vi "Merge Call Library Errors.vi"(4 "Library Call Returned Error":errorcluster, 6 "Error Code":i32(ring) items=["No Error", "mArgsErr", "mZoneErr", "mFullErr"], 8 "error in":errorcluster) -> (0 "error out":errorcluster)   [LabVIEW 2020, in "ase.lvlib" / "ase.lvclass"]
doc: "Combine Call Library Function Node Errors and Error Codes."
uses:
  ase.lvclass
  ase.lvclass/ase.ctl
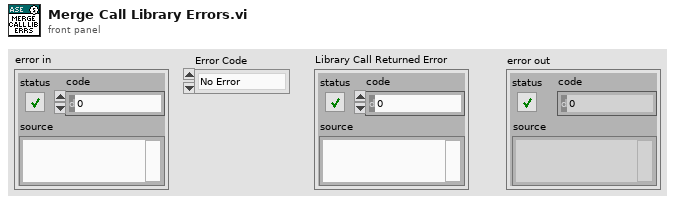
[diagram p1: front panel]
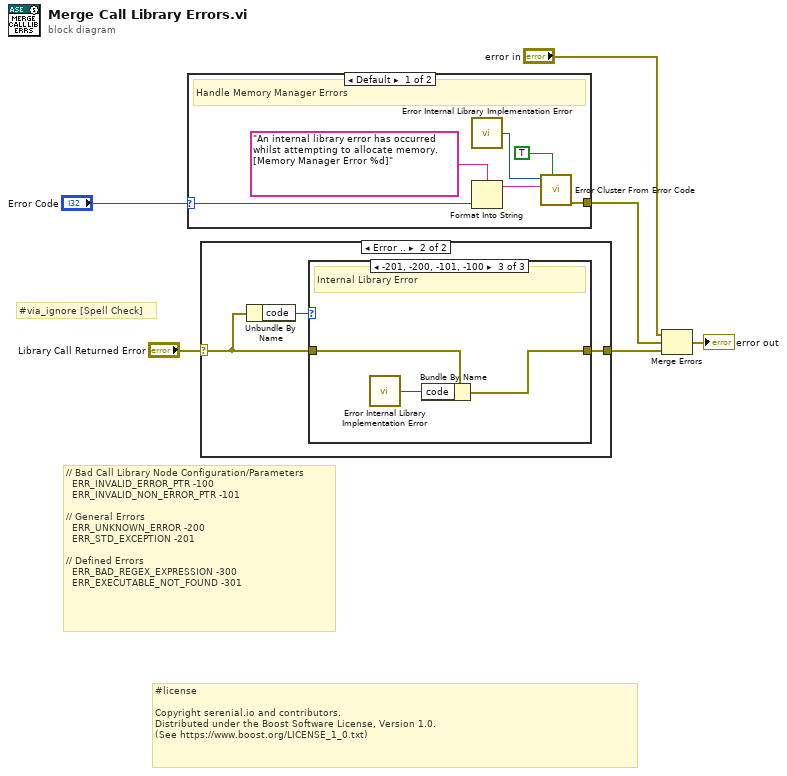
[diagram p0: block diagram]
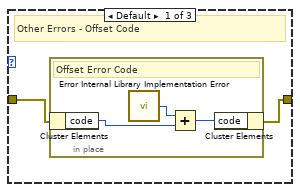
[diagram p3: hidden frame]
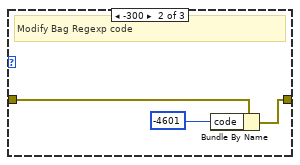
[diagram p4: hidden frame]
diagram:
  # "#via_ignore [Spell Check]"
  # "#license\n\nCopyright serenial.io and contributors.\nDistributed under the Boost Software License, Version 1.0.\n(See https://www.boost.org/LICENSE_1_0.txt)"
  # "// Bad Call Library Node Configuration/Parameters\n  ERR_INVALID_ERROR_PTR -100\n  ERR_INVALID_NON_ERROR_PTR -101\n\n// General Errors\n  ERR_UNKNOWN_ERROR -200\n  ERR_STD_EXCEPTION -201\n\n// Defined Errors\n  ERR_BAD_REGEX_EXPRESSION -300\n  ERR_EXECUTABLE_NOT_FOUND -301"
  n1 = case shown="Default" "Error Code" {
    selector: "Error Code" -> [w9 _]
    tunnel: [w12 _] -> w2
    frame Default {
      # "Handle Memory Manager Errors"
      n2 = call "Error Internal Library Implementation Error.vi"() -> ("Error Code"=w8:i32)
      n3 = Format Into String(format string="An internal library error has occurred whilst attempting to allocate memory. [Memory Manager Error %d]" ("error message (\"\")"), w9) -> (resulting string=w10:string)  [unwired: 2 in, 1 out]
      n4 = call <vilib>:"Error Cluster From Error Code.vi"("show call chain? (False)"=TRUE, "error message (\"\")"=w10, "error code (0)"=w8) -> ("error out"=w12:errorcluster)  [unwired: 6 in]
    }
    frame 0 {
      # "No Error"
    }
  }
  n5 = case shown="Error .." "Library Call Returned Error" {
    selector: "Library Call Returned Error" -> [w13 w15]
    tunnel: [w13 w16] -> w1
    frame No Error {
    }
    frame Error {
      n6 = Unbundle By Name(w15) -> ("code"=w14:i32)
      n7 = case shown="-201, -200, -101, -100" w14 {
        tunnel: [w17 w24 w26] -> w16
        tunnel: w15 -> [w18 w23 w27]
        frame Default {
          # "Other Errors - Offset Code"
          n8 = in-place "In Place Element Structure" {
            # "Offset Error Code"
            n9 = in-place-cluster #1 ("Unbundle / Bundle Elements")(w18) -> ("code"=w21:i32)
            n10 = call "Error Internal Library Implementation Error.vi"() -> ("Error Code"=w19:i32)
            n11 = Add(x=w19, y=w21) -> (x+y=w20:i32)
            n12 = in-place-cluster #1 ("Unbundle / Bundle Elements")("code"=w20) -> (w17:errorcluster)
          }
        }
        frame -300 {
          # "Modify Bag Regexp code"
          n13 = Bundle By Name(cluster=w23, "code"=-4601 ("y")) -> (w24:errorcluster)
        }
        frame -201, -200, -101, -100 {
          # "Internal Library Error"
          n14 = call "Error Internal Library Implementation Error.vi"() -> ("Error Code"=w25:i32)
          n15 = Bundle By Name(cluster=w27, "code"=w25) -> (w26:errorcluster)
        }
      }
    }
  }
  n16 = Merge Errors("error in", w2, w1) -> (→"error out":errorcluster)
